vi "_XNET Convert Time U64 100ns to LV.vi"(3 "Time U64 100ns":u64) -> (1 "Time LV":timestamp)   [LabVIEW 2018]
uses:
  nixlvapi.dll
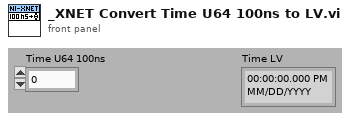
[diagram p1: front panel]
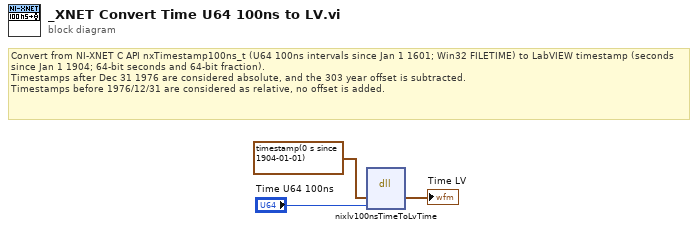
[diagram p0: block diagram]
diagram:
  # "Convert from NI-XNET C API nxTimestamp100ns_t (U64 100ns intervals since Jan 1 1601; Win32 FILETIME) to LabVIEW timestamp (seconds since Jan 1 1904; 64-bit seconds and 64-bit fraction).\nTimestamps after Dec 31 1976 are considered absolute, and the 303 year offset is subtracted.\nTimestamps before 1976/12/31 are considered as relative, no offset is added."
  n1 = dll-call lib="nixlvapi.*" fn="nixlv100nsTimeToLvTime" label="Call Library"("lvTime"=timestamp(0 s since 1904-01-01) ("Time LV"), "cTime"="Time U64 100ns") -> ("lvTime"=→"Time LV":timestamp)  [unwired: 4 in, 3 out]
